vi "Untitled 3.vi"() -> ()   [LabVIEW 2015]
uses:
  Controls/Sample Push Control Enumerator.ctl
panel:
  in  "Sample Push Control 16":T1
  in  "Sample Push Control 15":T1
  in  "Sample Push Control 14":T1
  in  "Sample Push Control 13":T1
  in  "Sample Push Control 12":T1
  in  "Sample Push Control 11":T1
  in  "Sample Push Control 10":T1
  in  "Sample Push Control 9":T1
  in  "Sample Push Control 8":T1
  in  "Sample Push Control 7":T1
  in  "Sample Push Control 6":T1
  in  "Sample Push Control 5":T1
  in  "Sample Push Control 4":T1
  in  "Sample Push Control 3":T1
  in  "Sample Push Control 2":T1
  in  "Sample Push Control":T1
  in  "Ring":u8(ring)
  out "Baratron 1":dbl(knob) scale=0.01..1000.0
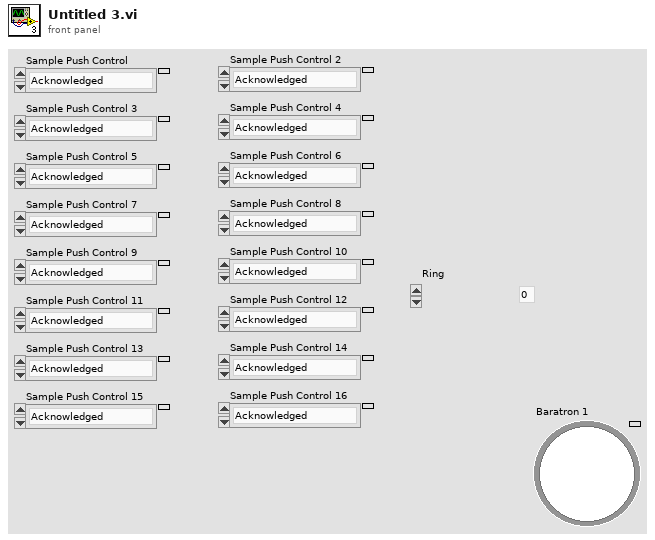
[diagram p1: front panel]
types:
  T1 = typedef "Sample Push Control Enumerator.ctl" = enum16{"Acknowledged", "Push", "Stash", "Abort", "Reset to Idle"}
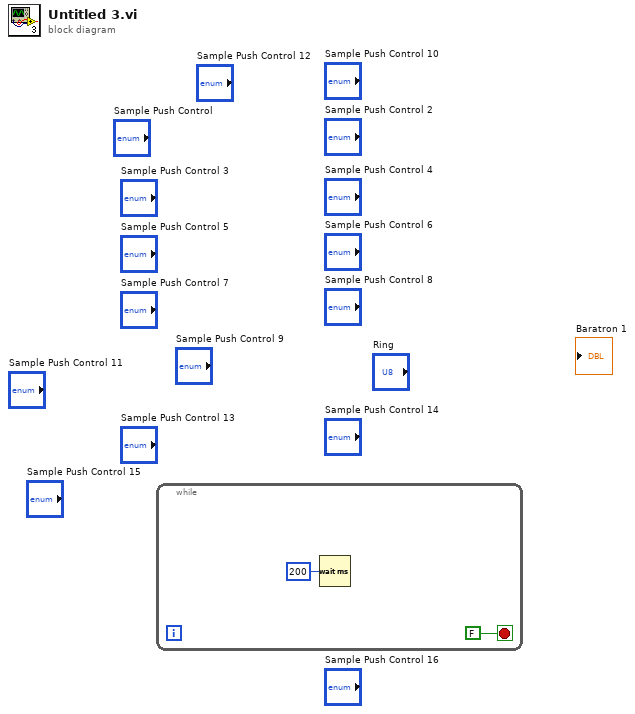
[diagram p0: block diagram]
diagram:
  n1 = while {
    stop <- FALSE stop-if-true
    n2 = Wait (ms)(milliseconds to wait=u32 200) -> ()  [unwired: 1 out]
  }
